vi "CalculateExpectedExtinctionIncludingDoublyChargeParticleCorrection.vi"(2 "refractive index, imaginary":sgl=0.1 step=0.01 format="%.3f", 3 "refractive index, real":sgl=1.3 step=0.01 format="%.3f", 4 "Extinction ExtinctionUncertainity Size parameter and Number ofS sizes":T1={"Extinction"=[], "Extinction Uncertainty"=[], "Size parameters"=[], "Number ofSizes"=0.0, "GeometricCrossSection"=[], "Wave Length"=0.0, "SMPS Sizes"=[], "Concentration"=[], "Double Charge Correction"=FALSE, "Extincation Factor"=1.0, "Diameter Factor"=1.0, "Diameter Offset"=0.0, "Extinction Factor Flag"=FALSE, "Diameter Factor Flag"=FALSE, "Diameter Offset Flag"=FALSE, "Sizes"=[], "ExtinctionOrAbsorptionOrScattering"=0} {"ExtinctionOrAbsorptionOrScattering" scale=0.0..2.0}) -> (0 "Expected Extinction graph":cluster{"Size parameters":dbl[], dbl[]}, 1 "Expected Extinction Cross Section":sgl[](array[numeric]))   [LabVIEW 2013]
uses:
  BaesDataTypeDefinition.ctl
  <vilib>/Analysis/baseanly.llb/Real Dot Product.vi
  <vilib>/imath/engines/lvmath2/RunTimeEngine/ErrorHandling/NIMS_Finalize Error.vi
  <vilib>/imath/engines/lvmath2/RunTimeEngine/Managers/WorkSpace/UID Generator.vi
  <vilib>/imath/engines/lvmath2/RunTimeEngine/Managers/SymbolTable/Clear UID.vi
  <vilib>/imath/engines/lvmath2/RunTimeEngine/NodeEndStatement/NIMS_NodeEndStatement_Output.vi
  <instcachedir>/0/NIMS_NodeEndStatement_Output_53EC0D466D134D7ABD903AC30B43404B.lvgen/NIMS_NodeEndStatement_Output_53EC0D466D134D7ABD903AC30B43404B_005.vi
  <vilib>/imath/engines/lvmath2/RunTimeEngine/RunTimeType/NIMS_RunTimeType_From StrictType (excl LVString).vi
  <instcachedir>/0/NIMS_RunTimeType_From StrictType (excl LVString)_4DEE718D6EB74582AA20236969C084FC.lvgen/NIMS_RunTimeType_From StrictType (excl LVString)_4DEE718D6EB74582AA20236969C084FC_000.vi
  <vilib>/imath/engines/lvmath2/RunTimeEngine/LocalVariableDefStatement/MC_LocalVariableDefStatement_Display.vi
  mie2.dll
  <vilib>/Analysis/NI_AALBase.lvlib
  <vilib>/imath/engines/lvmath2/RunTimeEngine/Managers/SymbolTable/NIMS_WorkSpace.lvlib
panel:
  out "totalscatter 3":sgl=3.7788873
  out "backscatter 3":sgl=8.098428
  out "<cos(theta)> 4":sgl=0.19839454
  out "extinction 3":sgl=1.6240653
  in  "angles (will compute\n2*angles-1 points from\n0...180 degrees)":u32=2
  out "totalscatter 2":sgl=3.7788873
  out "backscatter 2":sgl=8.098428
  out "<cos(theta)> 3":sgl=0.19839454
  out "extinction 2":sgl=1.6240653
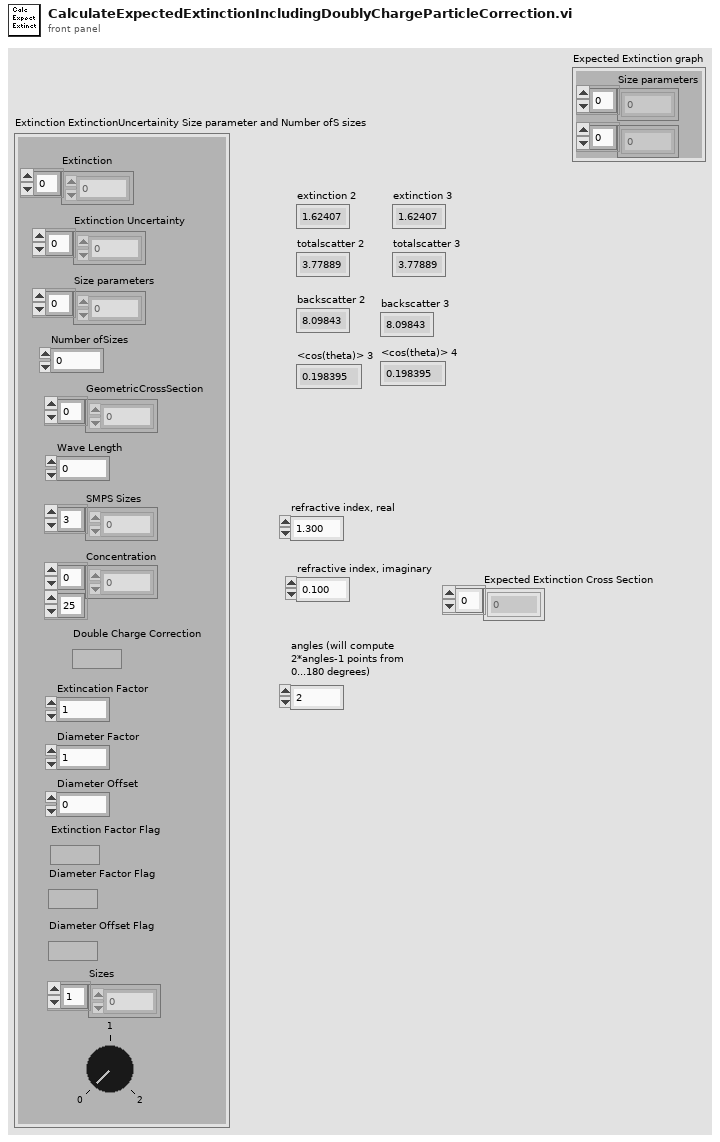
[diagram p1: front panel]
types:
  T1 = typedef "BaesDataTypeDefinition.ctl" = cluster{"Extinction":dbl[], "Extinction Uncertainty":dbl[], "Size parameters":dbl[], "Number ofSizes":dbl, "GeometricCrossSection":dbl[], "Wave Length":dbl, "SMPS Sizes":dbl[], "Concentration":dbl[][], "Double Charge Correction":bool, "Extincation Factor":dbl, "Diameter Factor":dbl, "Diameter Offset":dbl, "Extinction Factor Flag":bool, "Diameter Factor Flag":bool, "Diameter Offset Flag":bool, "Sizes":dbl[], "ExtinctionOrAbsorptionOrScattering":i8}
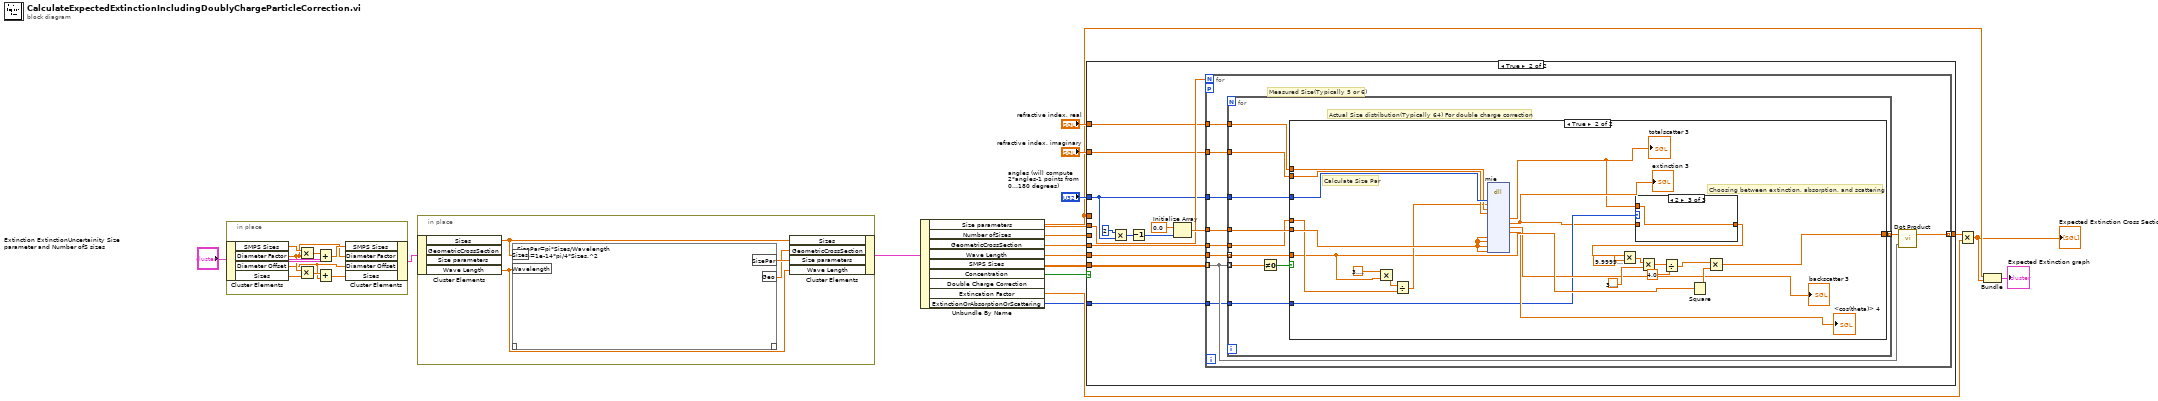
[diagram p0: block diagram]
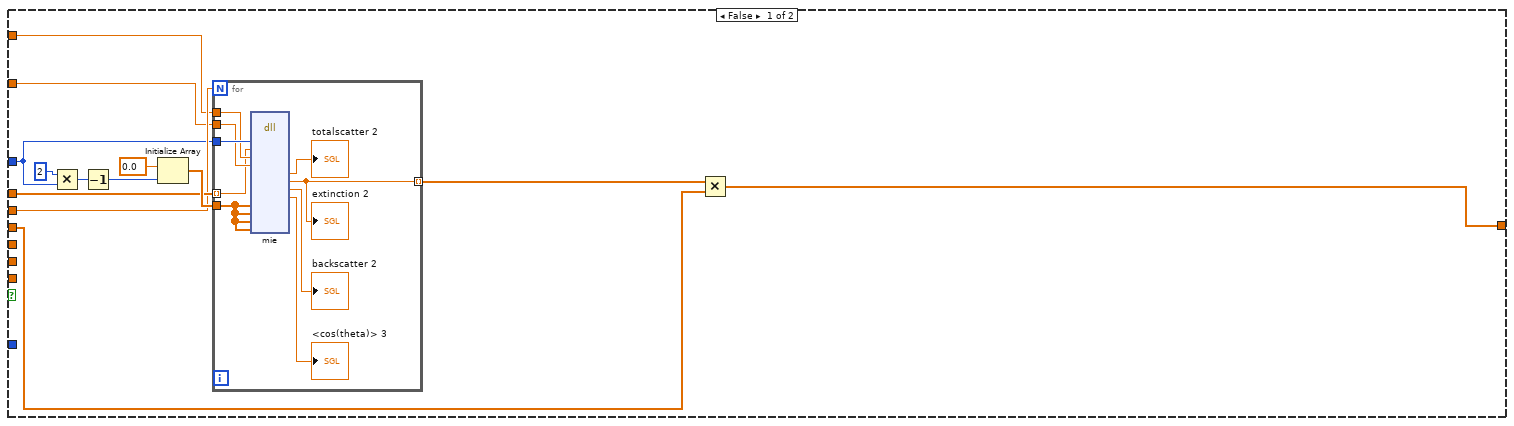
[diagram p2: hidden frame]
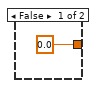
[diagram p3: hidden frame]
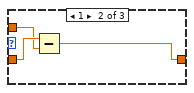
[diagram p5: hidden frame]
diagram:
  n1 = in-place {
    n2 = in-place-cluster #1("Extinction ExtinctionUncertainity Size parameter and Number ofS sizes") -> ("SMPS Sizes"=w26:dbl[], "Diameter Factor"=w22:dbl, "Diameter Offset"=w20:dbl, "Sizes"=w23:dbl[])
    n3 = Multiply(x=w26, y=w22) -> (x*y=w25:dbl[])
    n4 = Multiply(x=w22, y=w23) -> (x*y=w21:dbl[])
    n5 = Add(x=w25, y=w20) -> (x+y=w24:dbl[])
    n6 = Add(x=w21, y=w20) -> (x+y=w19:dbl[])
    n7 = in-place-cluster #1("SMPS Sizes"=w24, "Diameter Factor"=w22, "Diameter Offset"=w20, "Sizes"=w19) -> (w6:T1)
  }
  n8 = in-place {
    n9 = in-place-cluster #2(w6) -> ("Sizes"=w30:dbl[], "Wave Length"=w28:dbl)  [unwired: 2 out]
    n10 = mathscript code="SizePar=pi*Sizes/Wavelength\nGeo=1e-14*pi/4*Sizes.^2"("Sizes"=w30, "Wavelength"=w28) -> ("SizePar"=w29:dbl[], "Geo"=w27:dbl[])  [unwired: 1 in, 1 out]
    n11 = in-place-cluster #2("Sizes"=w30, "GeometricCrossSection"=w27, "Size parameters"=w29, "Wave Length"=w28) -> (w5:T1)
  }
  n12 = Unbundle By Name(w5) -> ("Size parameters"=w9:dbl[], "Number ofSizes"=w18:dbl, "GeometricCrossSection"=w17:dbl[], "Wave Length"=w11:dbl, "SMPS Sizes"=w12:dbl[], "Concentration"=w10:dbl[][], "Double Charge Correction"=w16:bool, "Extincation Factor"=w4:dbl, "ExtinctionOrAbsorptionOrScattering"=w1:i8)
  n13 = case shown="True" w16 {
    tunnel: w9 -> [w99 _]
    tunnel: w18 -> [w98 w122]
    tunnel: w17 -> [w96 _]
    tunnel: "angles (will compute\n2*angles-1 points from\n0...180 degrees)" -> [w95 w121]
    tunnel: "refractive index, imaginary" -> [w94 w120]
    tunnel: "refractive index, real" -> [w93 w119]
    tunnel: w12 -> [_ w118]
    tunnel: w11 -> [_ w117]
    tunnel: w10 -> [_ w116]
    tunnel: [w92 w115] -> w3
    tunnel: w1 -> [_ w114]
    frame False {
      n14 = Multiply(x=u32 2, y=w95) -> (x*y=w103:u32)
      n15 = Decrement(x=w103) -> (x-1=w101:u32)
      n16 = Initialize Array(sgl 0.0, w101) -> (w100:sgl[])
      n17 = for {
        N: w98 -> [_]
        tunnel: w100 -> [w111]
        tunnel: w95 -> [w110]
        tunnel: w93 -> [w109]
        tunnel: w94 -> [w108]
        tunnel: w99 -> [w107] mode=indexing
        tunnel: [w105] -> w97 mode=indexing
        n18 = dll-call lib="Z:/Downloads/Lior Segev Code Projects/RiRetrievalForLabview/mie2.dll" fn="mie"("angles"=w110, "x"=w107, "r"=w109, "i"=w108, "spol_real"=w111, "spol_imaginary"=w111, "ppol_real"=w111, "ppol_imaginary"=w111) -> ("totalscatter"=→"totalscatter 2":sgl, "extinction"=w105:sgl, "backscatter"=→"backscatter 2":sgl, "<cos(theta)>"=→"<cos(theta)> 3":sgl)  [unwired: 16 in, 2 out]
        "extinction 2" <- w105
      }
      n19 = Multiply(x=w97, y=w96) -> (x*y=w92:dbl[])
    }
    frame True {
      n20 = Multiply(x=u32 2, y=w121) -> (x*y=w126:u32)
      n21 = Decrement(x=w126) -> (x-1=w124:u32)
      n22 = Initialize Array(sgl 0.0, w124) -> (w123:sgl[])
      n23 = for {
        N: w122 -> [_]
        tunnel: w123 -> [w137]
        tunnel: w121 -> [w136]
        tunnel: w119 -> [w135]
        tunnel: w120 -> [w134]
        tunnel: w118 -> [w133]
        tunnel: w117 -> [w132]
        tunnel: w116 -> [w130] mode=indexing
        tunnel: [w131] -> w115 mode=indexing
        workers-P: _ -> [_]
        tunnel: w114 -> [w128]
        # "Measured Size(Typically 5 or 6)"
        n24 = for {
          tunnel: w137 -> [w147]
          tunnel: w136 -> [w146]
          tunnel: w135 -> [w145]
          tunnel: w134 -> [w144]
          tunnel: w133 -> [w139] mode=indexing
          tunnel: w132 -> [w142]
          tunnel: w130 -> [w141] mode=indexing
          tunnel: [w140] -> w129 mode=indexing
          tunnel: w128 -> [w138]
          # "Actual Size distribution(Typically 64) For double charge correction"
          n25 = Not Equal To 0?(x=w141) -> (x != 0?=w143:bool)
          n26 = case shown="True" w143 {
            tunnel: w147 -> [_ w171]
            tunnel: w146 -> [_ w170]
            tunnel: w145 -> [_ w169]
            tunnel: w144 -> [_ w168]
            tunnel: w139 -> [_ w157]
            tunnel: w142 -> [_ w165]
            tunnel: [0.0 ("ExtCross") w155] -> w140
            tunnel: w138 -> [_ w152]
            frame False {
            }
            frame True {
              # "Choosing between extinction, absorption, and scattering"
              # "Calculate Size Par"
              n27 = Multiply(x=3.141592653589793, y=w157) -> (x*y=w166:dbl)
              n28 = Divide(x=w166, y=w165) -> (x/y=w164:dbl)
              n29 = dll-call lib="Z:/Downloads/Lior Segev Code Projects/RiRetrievalForLabview/mie2.dll" fn="mie"("angles"=w170, "x"=w164, "r"=w169, "i"=w168, "spol_real"=w171, "spol_imaginary"=w171, "ppol_real"=w171, "ppol_imaginary"=w171) -> ("totalscatter"=w149:sgl, "extinction"=w151:sgl, "backscatter"=→"backscatter 3":sgl, "<cos(theta)>"=→"<cos(theta)> 4":sgl)  [unwired: 16 in, 2 out]
              "totalscatter 3" <- w149
              "extinction 3" <- w151
              n30 = case shown="2" w152 {
                tunnel: w151 -> [w172 w175 _]
                tunnel: [w172 w173 w176] -> w150
                tunnel: w149 -> [_ w174 w176]
                frame 0, Default {
                }
                frame 1 {
                  n31 = Subtract(x=w175, y=w174) -> (x-y=w173:sgl)
                }
                frame 2 {
                }
              }
              n32 = Multiply(x=w150, y=sgl 1e-14) -> (x*y=w163:sgl)
              n33 = Multiply(x=w163, y=3.141592653589793) -> (x*y=w160:dbl)
              n34 = Divide(x=w160, y=4.0) -> (x/y=w158:dbl)
              n35 = Square(x=w157) -> (x^2=w156:dbl)
              n36 = Multiply(x=w158, y=w156) -> (x*y=w155:dbl)
            }
          }
        }
        n37 = call-poly <vilib>:"Dot Product.vi"("Y Vector"=w130, "X Vector"=w129) -> ("X * Y"=w131:dbl)  [unwired: 1 out]
      }
    }
  }
  n38 = Multiply(x=w3, y=w4) -> (x*y=w2:dbl[])
  "Expected Extinction Cross Section" <- w2
  n39 = Bundle("Size parameters"=w9, w2) -> (→"Expected Extinction graph":cluster{"Size parameters":dbl[], dbl[]})  [unwired: 1 in]
